vi "AddSongToPlaylist.vi"(0 "reference in":refnum<class "MusicPlayer.lvclass">, 7 "File Path":path, 11 "Error In":errorcluster) -> (4 "reference out":refnum<class "MusicPlayer.lvclass">, 15 "Error Out":errorcluster)   [LabVIEW 2022 SP3, in "MusicPlayer.lvclass"]
uses:
  MusicPlayer.lvclass
  MusicPlayer.lvclass/MusicPlayer.ctl
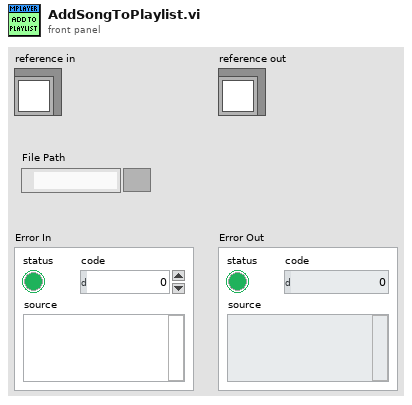
[diagram p1: front panel]
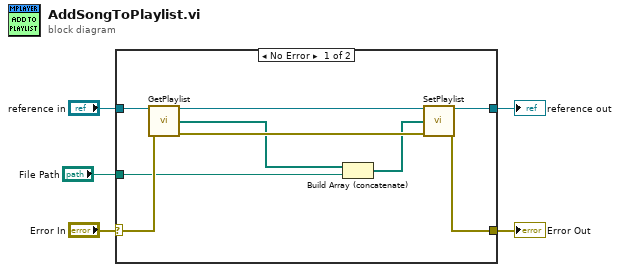
[diagram p0: block diagram]
diagram:
  n1 = case shown="No Error" "Error In" {
    selector: "Error In" -> [w9 w16]
    tunnel: [w13 w16] -> w4
    tunnel: [w11 w15] -> w2
    tunnel: "reference in" -> [w10 w15]
    tunnel: "File Path" -> [w6 _]
    frame No Error {
      n2 = call "GetPlaylist.vi"("reference in"=w10, "Error In"=w9) -> ("reference out"=w12:refnum<class "MusicPlayer.lvclass">, "Playlist"=w8:path[], "Error Out"=w14:errorcluster)  [unwired: 11 in]
      n3 = Build Array (concatenate)(w8, w6) -> (w7:path[])
      n4 = call "SetPlaylist.vi"("reference in"=w12, "Playlist"=w7, "Error In"=w14) -> ("reference out"=w11:refnum<class "MusicPlayer.lvclass">, "Error Out"=w13:errorcluster)  [unwired: 11 in]
    }
    frame Error {
    }
  }
  "Error Out" <- w4
  "reference out" <- w2
